vi "Read Delays.vi"(8 "error in (no error)":errorcluster, 11 "Gif Parent in":refnum<class "Gif Parent.lvclass">) -> (0 "error out":errorcluster, 2 "Delays":i32[](array[numeric]), 3 "Gif Parent out":refnum<class "Gif Parent.lvclass">)   [LabVIEW 2019, in "Pop-Up.lvlib" / "Gif Parent.lvclass"]
doc: "read the delay array for the gif frames"
uses:
  Gif Parent.lvclass
  Gif Parent.lvclass/Gif Parent.ctl
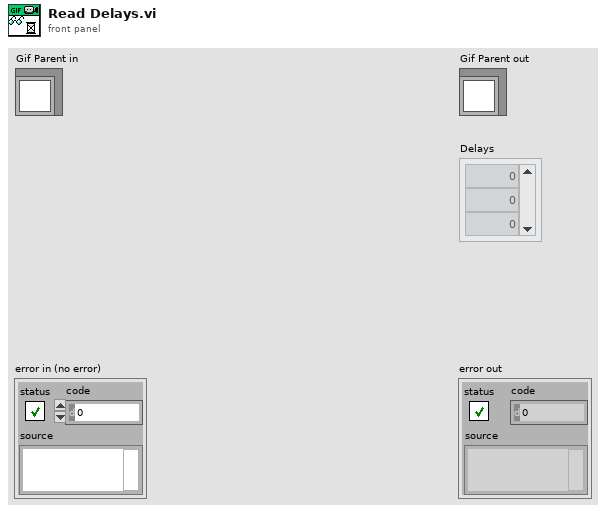
[diagram p1: front panel]
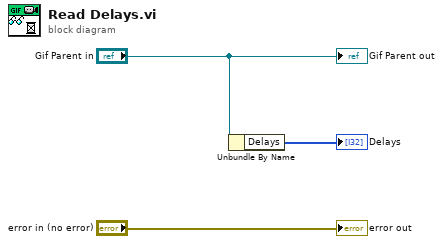
[diagram p0: block diagram]
diagram:
  n1 = Unbundle By Name("Gif Parent in") -> ("Delays"=→"Delays":i32[])
  "error out" <- "error in (no error)"
  "Gif Parent out" <- "Gif Parent in"
